vi "glueAlignPinInsert_Stereo.vi"() -> ()   [LabVIEW 2015]
uses:
  GlobalPath.vi
  GlobalData.vi
  GlobalVi.vi
panel:
  in  "ptfe 33":bool caption="Remove the electroerosion pin (stereo+eta) and the precision rod (eta only)"
  in  "ptfe 10":bool caption="Place and screw the blocking plate to the vertical positioning tool to keep the pin orthogonality during the curing of the glue"
  in  "ptfe 40":bool caption="Insert the electroerosition pin in the slotted insert and the precision rod in the circular insert"
  in  "ptfe 38":bool caption="Check the planarity of the tool with the gauge machine"
  in  "ptfe 37":bool caption="Tighten the three screws to block the vertical positioning tool in place"
  in  "ptfe 35":bool caption="Position the vertical positioning tool on the reference plate against with its positioning pins"
  in  "ptfe 34":bool caption="Deposit the glue on the stainless steel slotted and circular insert groove"
  in  "ptfe 32":bool caption="Position the inserts in the dedicated hole on the panel"
  in  "ptfe 26":bool caption="Position the panel on the table"
  in  "ptfe 25":bool caption="Move the panel away from the table"
  in  "ptfe 24":bool caption="Lift the panel from the table"
  in  "ptfe 23":bool caption="Switch on the vacuum on the machine"
  in  "ptfe 22":bool caption="Lower the machine on the panel"
  in  "ptfe 21":bool caption="Move the rotating machine on top of the panel"
  in  "Done ?":bool
  in  "ptfe 20":bool caption="Wait 24h for the glue to cure"
  in  "ptfe 19":bool caption="Apply the reinforcing washer"
  in  "ptfe 18":bool caption="Deposit the glue on the emerging part of the alignment pins (stereo only)/inserts (one for stereo, two for eta) using a thin needle"
  in  "ptfe 17":bool caption="Rotate the panel so that it's back side is up"
  in  "ptfe 16":bool caption="Switch off the vacuum"
  in  "ptfe 15":bool caption="Remove the three vertical positioning tools, blocking plates and positioning pins"
  in  "ptfe 14":bool caption="Wait 24h for the glue to cure"
  in  "ptfe 2":bool caption="Check that the vacuum is on"
  # "Gluing of Alignment Pin/Insert"
  # "ETA PANEL \nINSTRUCTIONS"
  # "GLUING OF THE SLOTTED BRASS AND CIRCULAR BRASS INSERT"
  # "Add info on enumeration"
  # "COMMON STEPS FOR\nBOTH PANELS"
  # "GLUE CURING OF THE TWO PINS AND INSERT"
  # "GLUING OF REINFORCING WASHER ON PANEL BACK SIDE"
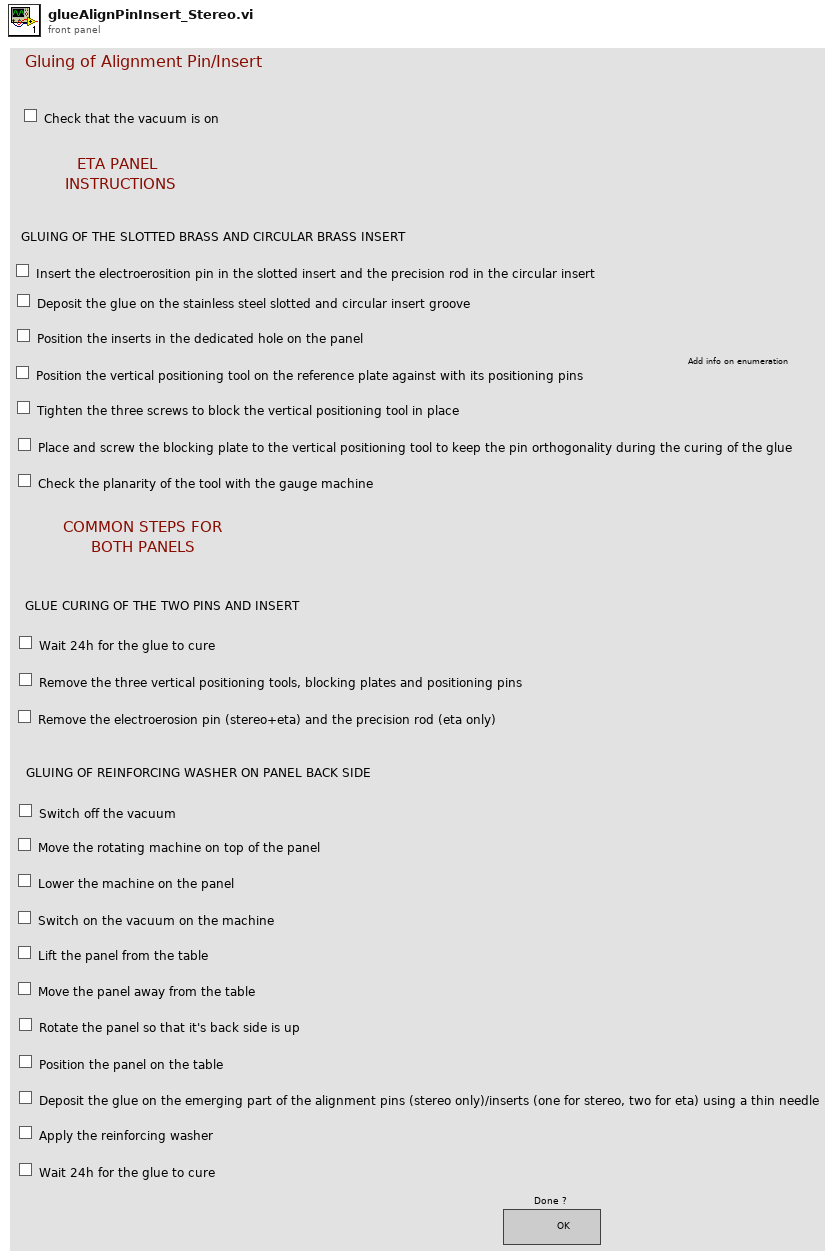
[diagram p1: front panel]
types:
  T1 = enum16{"open", "replace", "create", "open or create", "replace or create", "replace or create with confirmation"}
  T2 = enum32{"Bad", "Idle", "Run top level", "Running"}
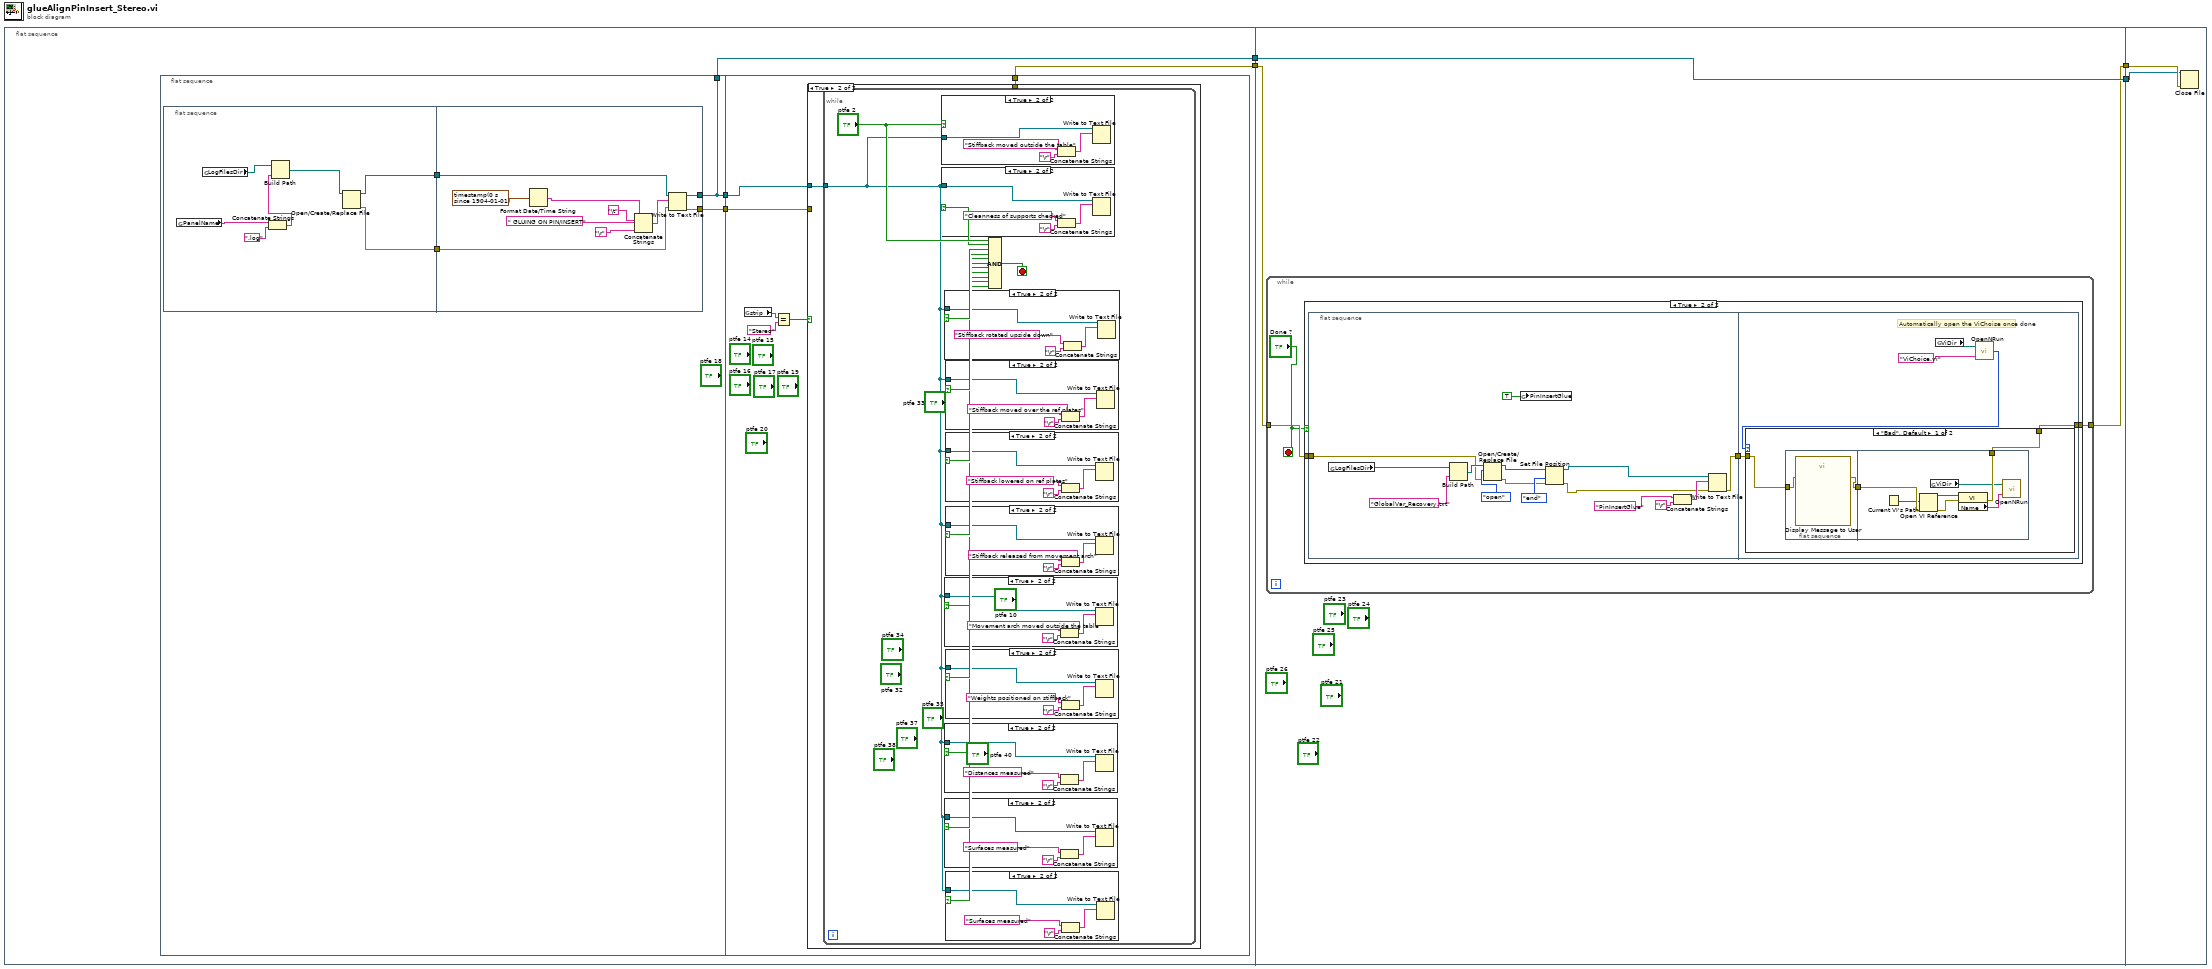
[diagram p0: block diagram]
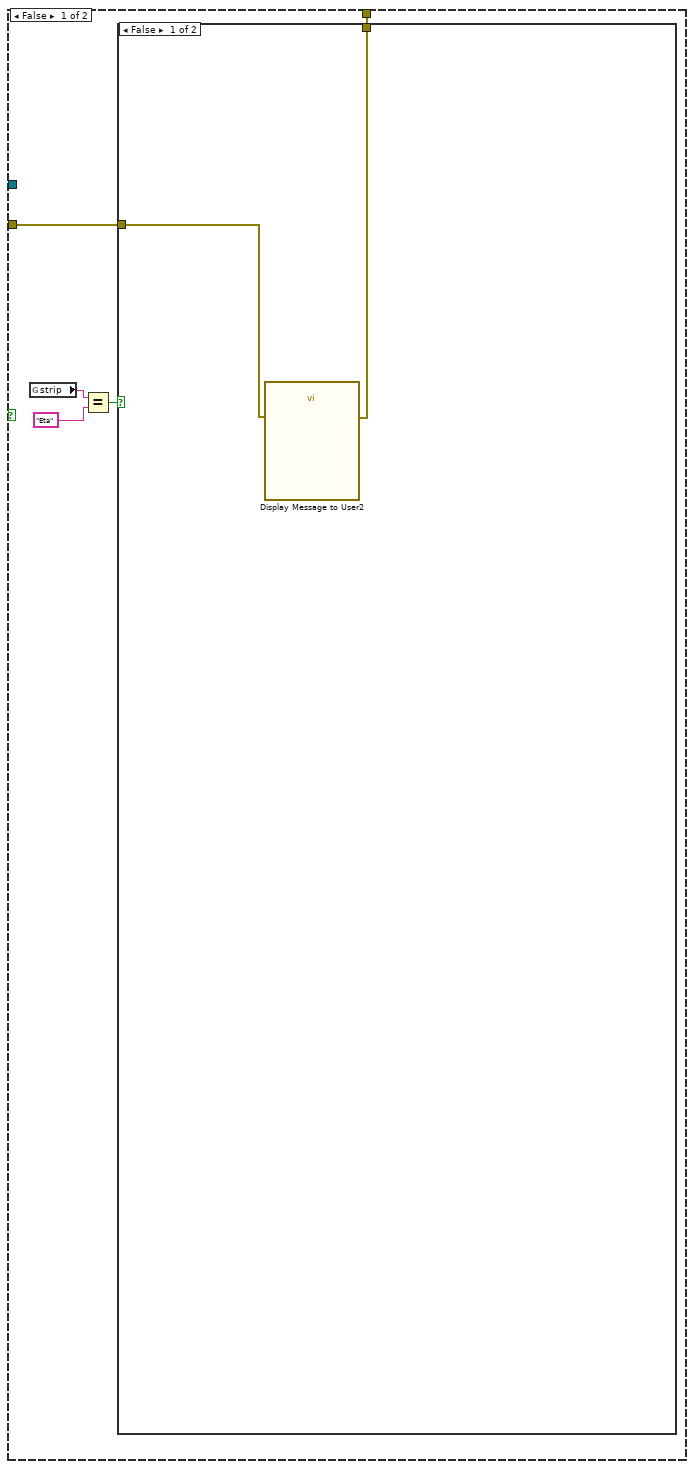
[diagram p2: hidden frame]
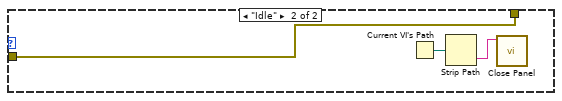
[diagram p16: hidden frame]
diagram:
  n1 = flat-sequence {
    tunnel: [w5] -> w3
    tunnel: [w7] -> w2
    tunnel: [w101] -> w4
    tunnel: w3 -> [w102]
    tunnel: w2 -> [w103]
    tunnel: [w103] -> w1
    tunnel: w4 -> [w147]
    tunnel: w1 -> [w146]
    frame #0 {
      n2 = flat-sequence {
        tunnel: [w11] -> w8
        tunnel: [w11] -> w7
        tunnel: [w9] -> w6
        tunnel: w8 -> [w35]
        tunnel: w6 -> [w31]
        tunnel: [w30] -> w5
        frame #0 {
          n3 = flat-sequence {
            tunnel: [w14] -> w12
            tunnel: [w13] -> w10
            tunnel: w12 -> [w23]
            tunnel: [w22] -> w11
            tunnel: [w21] -> w9
            tunnel: w10 -> [w20]
            frame #0 {
              n4 = global read "GlobalData.vi" "PanelName"() -> (w17:string)
              n5 = global read "GlobalPath.vi" "LogFilesDir"() -> (w19:path)
              n6 = Concatenate Strings(w17, ".log") -> (w16:string)
              n7 = Build Path(base path=w19, name or relative path=w16) -> (appended path=w15:path)
              n8 = Open/Create/Replace File(file path (use dialog)=w15) -> (refnum out=w14:refnum<file>, error out=w13:errorcluster)  [unwired: 5 in, 1 out]
            }
            frame #1 {
              n9 = Format Date/Time String(seconds (now)=timestamp(0 s since 1904-01-01)) -> (date/time string=w26:string)  [unwired: 2 in]
              n10 = Concatenate Strings(w26, "\t", " GLUING ON PIN/INSERT", "\r") -> (w24:string)
              n11 = Write to Text File(file (use dialog)=w23, text=w24, error in=w20) -> (refnum out=w22:refnum<file>, error out=w21:errorcluster)  [unwired: 1 in, 1 out]
            }
          }
        }
        frame #1 {
          n12 = global read "GlobalData.vi" "strip"() -> (w34:string)
          n13 = Equal?(x=w34, y="Stereo") -> (x = y?=w32:bool)
          n14 = case shown="True" w32 {
            tunnel: w35 -> [_ w43]
            tunnel: w31 -> [w37 _]
            tunnel: [w36 _] -> w30
            frame False {
              n15 = global read "GlobalData.vi" "strip"() -> (w40:string)
              n16 = Equal?(x=w40, y="Eta") -> (x = y?=w38:bool)
              n17 = case shown="False" w38 {
                tunnel: w37 -> [w42 _]
                tunnel: [w41 _] -> w36
                frame False {
                  n18 = call "Display Message to User2"("error in (no error)"=w42) -> ("error out"=w41:errorcluster)  [unwired: 9 in, 1 out]
                }
                frame True {
                }
              }
            }
            frame True {
              n19 = while {
                tunnel: w43 -> [w45]
                stop <- w56 stop-if-true
                n20 = case shown="True" "ptfe 2" {
                  tunnel: w45 -> [_ w97]
                  frame False {
                  }
                  frame True {
                    n21 = Concatenate Strings("Stiffback moved outside the table", "\r") -> (w100:string)
                    n22 = Write to Text File(file (use dialog)=w97, text=w100) -> ()  [unwired: 2 in, 3 out]
                  }
                }
                n23 = case shown="True" w54 {
                  tunnel: w45 -> [_ w93]
                  frame False {
                  }
                  frame True {
                    n24 = Concatenate Strings("Cleanness of supports checked", "\r") -> (w96:string)
                    n25 = Write to Text File(file (use dialog)=w93, text=w96) -> ()  [unwired: 2 in, 3 out]
                  }
                }
                n26 = case shown="True" w46 {
                  tunnel: w45 -> [_ w61]
                  frame False {
                  }
                  frame True {
                    n27 = Concatenate Strings("Movement arch moved outside the table", "\r") -> (w64:string)
                    n28 = Write to Text File(file (use dialog)=w61, text=w64) -> ()  [unwired: 2 in, 3 out]
                  }
                }
                n29 = case shown="True" w48 {
                  tunnel: w45 -> [_ w69]
                  frame False {
                  }
                  frame True {
                    n30 = Concatenate Strings("Distances measured", "\r") -> (w72:string)
                    n31 = Write to Text File(file (use dialog)=w69, text=w72) -> ()  [unwired: 2 in, 3 out]
                  }
                }
                n32 = case shown="True" w47 {
                  tunnel: w45 -> [_ w65]
                  frame False {
                  }
                  frame True {
                    n33 = Concatenate Strings("Surfaces measured", "\r") -> (w68:string)
                    n34 = Write to Text File(file (use dialog)=w65, text=w68) -> ()  [unwired: 2 in, 3 out]
                  }
                }
                n35 = case shown="True" w44 {
                  tunnel: w45 -> [_ w57]
                  frame False {
                  }
                  frame True {
                    n36 = Concatenate Strings("Surfaces measured", "\r") -> (w60:string)
                    n37 = Write to Text File(file (use dialog)=w57, text=w60) -> ()  [unwired: 2 in, 3 out]
                  }
                }
                n38 = Compound Arithmetic op=AND("ptfe 2", w54, w48, w47, w46, w44) -> (w56:bool, w53:bool, w52:bool, w51:bool, w50:bool, w49:bool)
                n39 = case shown="True" w53 {
                  tunnel: w45 -> [_ w89]
                  frame False {
                  }
                  frame True {
                    n40 = Concatenate Strings("Stiffback rotated upside down", "\r") -> (w92:string)
                    n41 = Write to Text File(file (use dialog)=w89, text=w92) -> ()  [unwired: 2 in, 3 out]
                  }
                }
                n42 = case shown="True" w51 {
                  tunnel: w45 -> [_ w81]
                  frame False {
                  }
                  frame True {
                    n43 = Concatenate Strings("Stiffback lowered on ref plates", "\r") -> (w84:string)
                    n44 = Write to Text File(file (use dialog)=w81, text=w84) -> ()  [unwired: 2 in, 3 out]
                  }
                }
                n45 = case shown="True" w50 {
                  tunnel: w45 -> [_ w77]
                  frame False {
                  }
                  frame True {
                    n46 = Concatenate Strings("Stiffback released from movement arch", "\r") -> (w80:string)
                    n47 = Write to Text File(file (use dialog)=w77, text=w80) -> ()  [unwired: 2 in, 3 out]
                  }
                }
                n48 = case shown="True" w49 {
                  tunnel: w45 -> [_ w73]
                  frame False {
                  }
                  frame True {
                    n49 = Concatenate Strings("Weights positioned on stiffback", "\r") -> (w76:string)
                    n50 = Write to Text File(file (use dialog)=w73, text=w76) -> ()  [unwired: 2 in, 3 out]
                  }
                }
                n51 = case shown="True" w52 {
                  tunnel: w45 -> [_ w85]
                  frame False {
                  }
                  frame True {
                    n52 = Concatenate Strings("Stiffback moved over the ref plates", "\r") -> (w88:string)
                    n53 = Write to Text File(file (use dialog)=w85, text=w88) -> ()  [unwired: 2 in, 3 out]
                  }
                }
              }
            }
          }
        }
      }
    }
    frame #1 {
      n54 = while {
        tunnel: [w106] -> w101
        tunnel: w102 -> [w105]
        stop <- "Done ?" stop-if-true
        n55 = case shown="True" "Done ?" {
          tunnel: [w107 w110] -> w106
          tunnel: w105 -> [w107 w109]
          frame False {
          }
          frame True {
            n56 = flat-sequence {
              tunnel: w109 -> [w114]
              tunnel: [w113] -> w108
              tunnel: [w127] -> w110
              tunnel: w108 -> [w126]
              frame #0 {
                n57 = global read "GlobalPath.vi" "LogFilesDir"() -> (w111:path)
                n58 = Build Path(base path=w111, name or relative path="GlobalVar_Recovery.txt") -> (appended path=w123:path)
                n59 = Open/Create/Replace File(file path (use dialog)=w123, error in=w114, operation (0:open)=T1."open") -> (refnum out=w119:refnum<file>, error out=w120:errorcluster)  [unwired: 3 in, 1 out]
                n60 = global write "GlobalVi.vi" "PinInsertGlue"(TRUE) -> ()
                n61 = Set File Position(refnum=w119, from (0:start)=enum16{"start", "end", "current"}."end", error in=w120) -> (refnum out=w116:refnum<file>, error out=w115:errorcluster)  [unwired: 1 in]
                n62 = Concatenate Strings("PinInsertGlue", "\r") -> (w118:string)
                n63 = Write to Text File(file (use dialog)=w116, text=w118, error in=w115) -> (error out=w113:errorcluster)  [unwired: 1 in, 2 out]
              }
              frame #1 {
                # "Automatically open the ViChoise once done"
                n64 = global read "GlobalPath.vi" "ViDir"() -> (w130:path)
                n65 = call "OpenNRun.vi"("VI name"="ViChoice.vi", "ViDirPath"=w130) -> ("Execution:State"=w129:T2)
                n66 = case shown="\"Bad\", Default" w129 {
                  tunnel: [w131 w143] -> w127
                  tunnel: w126 -> [w132 w143]
                  frame "Bad", Default {
                    n67 = flat-sequence {
                      tunnel: w132 -> [w135]
                      tunnel: [w134] -> w133
                      tunnel: [w139] -> w131
                      tunnel: w133 -> [w138]
                      frame #0 {
                        n68 = call "Display Message to User"("error in (no error)"=w135) -> ("error out"=w134:errorcluster)  [unwired: 9 in, 1 out]
                      }
                      frame #1 {
                        n69 = Current VI's Path() -> (path=w136:path)
                        n70 = Open VI Reference(vi path=w136, error in (no error)=w138) -> (vi reference=w142:refnum<vi>, error out=w141:errorcluster)  [unwired: 4 in]
                        n71 = global read "GlobalPath.vi" "ViDir"() -> (w137:path)
                        n72 = property class="VI"(reference=w142, error in=w141) -> (error out=w139:errorcluster, "Name"=w140:string)  [unwired: 1 out]
                        n73 = call "OpenNRun.vi"("VI name"=w140, "ViDirPath"=w137) -> ()  [unwired: 1 out]
                      }
                    }
                  }
                  frame "Idle" {
                    n74 = Current VI's Path() -> (path=w144:path)
                    n75 = Strip Path(path=w144) -> (name=w145:string)  [unwired: 1 out]
                    n76 = call <vilib>:"Close Panel.vi"("VI name"=w145) -> ()  [unwired: 10 in, 1 out]
                  }
                }
              }
            }
          }
        }
      }
    }
    frame #2 {
      n77 = Close File(refnum=w146, error in=w147) -> ()  [unwired: 2 out]
    }
  }
